vi "AppBar Variables.vi"(8 "error in (no error)":errorcluster, 11 "MainController in":refnum<class "MainController.lvclass">) -> (0 "error out":errorcluster, 1 "App Bar Height":i32=100, 2 "App Bar Peek Height":u32=24, 3 "MainController out":refnum<class "MainController.lvclass">)   [LabVIEW 2020, in "MainController.lvlib" / "MainController.lvclass"]
uses:
  MainController.lvclass
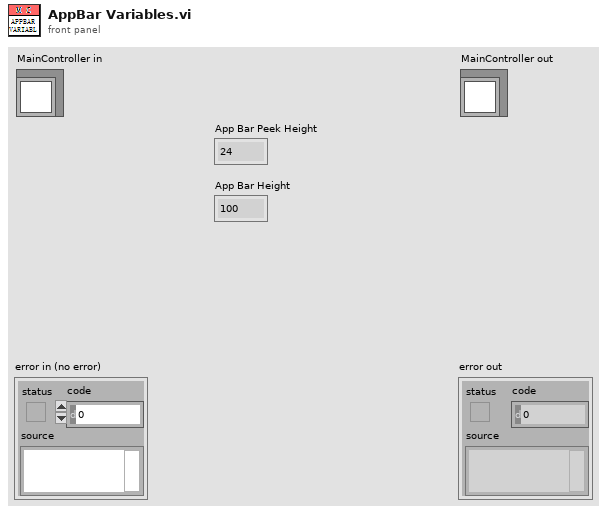
[diagram p1: front panel]
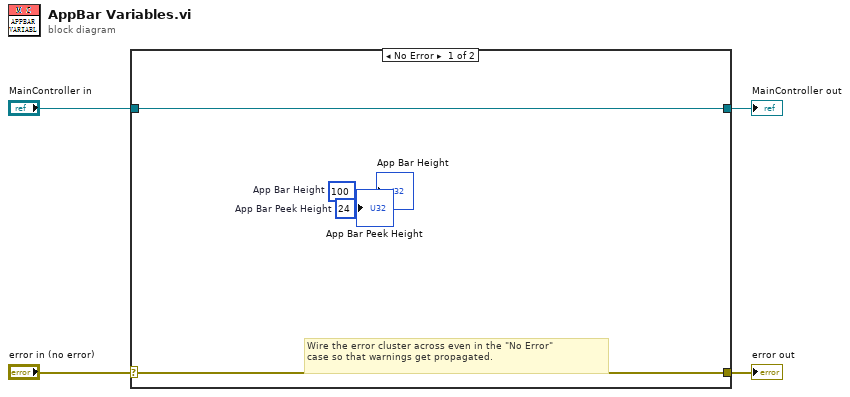
[diagram p0: block diagram]
diagram:
  n1 = case shown="No Error" "error in (no error)" {
    selector: "error in (no error)" -> [w7 w10]
    tunnel: [w7 w10] -> w3
    tunnel: [w8 w9] -> w1
    tunnel: "MainController in" -> [w8 w9]
    frame No Error {
      w5 = u32 24  # App Bar Peek Height
      w6 = 100  # App Bar Height
      # "Wire the error cluster across even in the \"No Error\"\ncase so that warnings get propagated."
      "App Bar Peek Height" <- w5
      "App Bar Height" <- w6
    }
    frame Error {
    }
  }
  "error out" <- w3
  "MainController out" <- w1
